vi "Power Output Test Parameters to Stimulus.vi"(10 "PO Test Parameters":T9={"Stimulus"={"Frequency Type"=enum."Band Edges", "Frequency Ranges"=[], "TX 1 Frequency (MHz)"={"Min"=0.0, "Max"=0.0}, "TX 2 Frequency (MHz)"={"Min"=0.0, "Max"=0.0}, "RX Frequency (MHz)"={"Min"=0.0, "Max"=0.0}, "Pad Model Number"="", "Pad Serial Number"="", "Pad Values"=[]}, "Measurement"={"DUT Port"=enum."Port 1", "Direction"=0, "Frequency Step Size"=0}, "Display"={"Frequency"={"Min"=-1.0, "Max"=-1.0}, "Power"={"Min"=-1, "Max"=-1}}, "Limit"={"Min Power (dBm)"=44.0}, "Calibration"={"Calibrated?"=FALSE}} {"Measurement"."Frequency Step Size" items=["0.2", "0.4", "1.0", "2.0", "4.0"]; "Measurement"."Direction" items=["Reverse", "Forward", "Auxiliary"]}) -> (2 "PIM Measurement Stimulus":T1={"Carrier Frequencies"={"C1 Freq, MHz"=0.0, "C2 Freq, MHz"=0.0}, "Carrier Powers"={"C1 Power,dBm"=0.0, "C2 Power, dBm"=0.0}, "Measurement Parameters"={"IM Order"=0, "Averaging"=1, "Direction"=0, "Enable ALC?"=FALSE, "Enable SingleIM?"=FALSE, "Display Units"=enum."dBm", "VA Hold?"=FALSE, "DUT PORT"=enum."Port 1"}, "Measurement Setup"={"Meas Type"=enum."Time", "TXStep"=0}} {"Measurement Setup"."TXStep" items=[".2", ".4", "1.0", "2.0"]; "Measurement Parameters"."Direction" items=["Reverse", "Forward", "Auxiliary"]; "Measurement Parameters"."IM Order" items=["3rd", "5th", "7th", "9th", "11th", "13th", "15th", "17th", "19th", "21st", "23rd", "25th", "27th", "29th", "31st", "33rd"]; "Measurement Parameters"."Averaging" items=["None", "Minimum", "Normal", "High", "Maximum"]})   [LabVIEW 2011]
uses:
  TypeDefs/Power Output Test Parameters.ctl
  TypeDefs/Power Output Stimulus Parameters.ctl
  TypeDefs/Power Output Measurement Parameters.ctl
  BPIMCore EXT/HW IO/DUTport.ctl
  BPIMCore EXT/HW IO/MeasMode.ctl
  BPIMCore EXT/HW IO/PIM Sweep Step Size.ctl
  TypeDefs/Power Output Display Parameters.ctl
  TypeDefs/Power Output Limit Parameters.ctl
  TypeDefs/Power Output Calibration State.ctl
  drivers/PIM/PIM Stimulus.ctl
  drivers/PIM/PIM Cmd Params.ctl
  BPIMCore EXT/HW IO/IMOrder.ctl
  BPIMCore EXT/HW IO/HW Averaging.ctl
  BPIMCore EXT/Display/display_unit_format.ctl
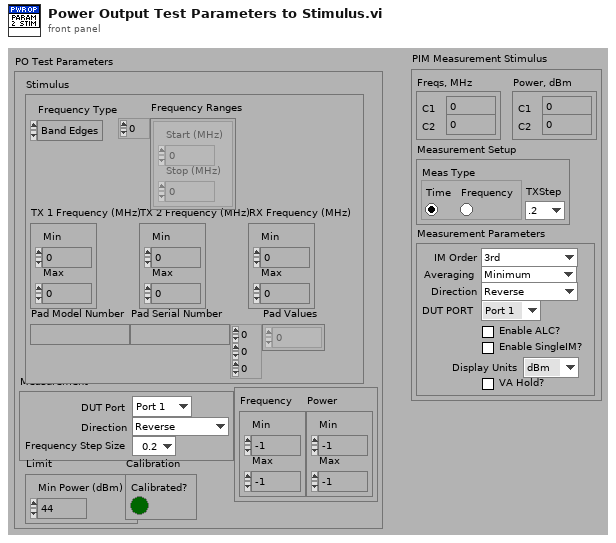
[diagram p1: front panel]
types:
  T1 = typedef "PIM Stimulus.ctl" = cluster{"Carrier Frequencies":cluster{"C1 Freq, MHz":dbl, "C2 Freq, MHz":dbl}, "Carrier Powers":cluster{"C1 Power,dBm":dbl, "C2 Power, dBm":dbl}, "Measurement Parameters":T2, "Measurement Setup":cluster{"Meas Type":enum32{"Time", "Frequency"}, "TXStep":T8}}
  T2 = typedef "PIM Cmd Params.ctl" = cluster{"IM Order":T3, "Averaging":T4, "Direction":T5, "Enable ALC?":bool, "Enable SingleIM?":bool, "Display Units":T6, "VA Hold?":bool, "DUT PORT":T7}
  T3 = typedef "IMOrder.ctl" = u8
  T4 = typedef "HW Averaging.ctl" = u16
  T5 = typedef "MeasMode.ctl" = u16
  T6 = typedef "display_unit_format.ctl" = enum16{"dBm", "dBc"}
  T7 = typedef "DUTport.ctl" = enum16{"Port 1", "Port 2"}
  T8 = typedef "PIM Sweep Step Size.ctl" = u16
  T9 = typedef "Power Output Test Parameters.ctl" = cluster{"Stimulus":T10, "Measurement":T11, "Display":T12, "Limit":T13, "Calibration":T14}
  T10 = typedef "Power Output Stimulus Parameters.ctl" = cluster{"Frequency Type":enum16{"Band Edges", "Custom"}, "Frequency Ranges":cluster{"Start (MHz)":dbl, "Stop (MHz)":dbl}[], "TX 1 Frequency (MHz)":cluster{"Min":dbl, "Max":dbl}, "TX 2 Frequency (MHz)":cluster{"Min":dbl, "Max":dbl}, "RX Frequency (MHz)":cluster{"Min":dbl, "Max":dbl}, "Pad Model Number":string, "Pad Serial Number":string, "Pad Values":dbl[][][]}
  T11 = typedef "Power Output Measurement Parameters.ctl" = cluster{"DUT Port":T7, "Direction":T5, "Frequency Step Size":T8}
  T12 = typedef "Power Output Display Parameters.ctl" = cluster{"Frequency":cluster{"Min":dbl, "Max":dbl}, "Power":cluster{"Min":i32, "Max":i32}}
  T13 = typedef "Power Output Limit Parameters.ctl" = cluster{"Min Power (dBm)":dbl}
  T14 = typedef "Power Output Calibration State.ctl" = cluster{"Calibrated?":bool}
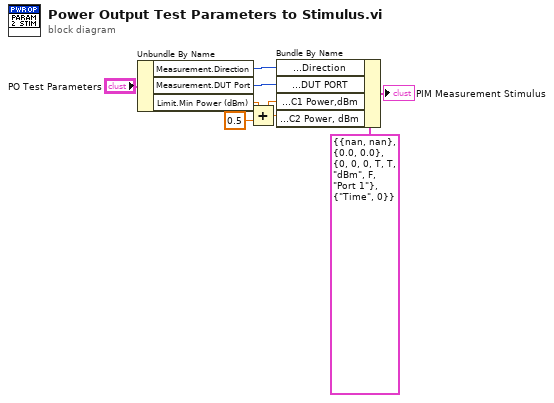
[diagram p0: block diagram]
diagram:
  n1 = Unbundle By Name("PO Test Parameters") -> ("Measurement.Direction"=w6:T5, "Measurement.DUT Port"=w4:T7, "Limit.Min Power (dBm)"=w2:dbl)
  n2 = Add(x=w2, y=0.5) -> (x+y=w1:dbl)
  n3 = Bundle By Name(cluster=T1 {"Carrier Frequencies"={"C1 Freq, MHz"=nan, "C2 Freq, MHz"=nan}, "Carrier Powers"={"C1 Power,dBm"=0.0, "C2 Power, dBm"=0.0}, "Measurement Parameters"={"IM Order"=0, "Averaging"=0, "Direction"=0, "Enable ALC?"=TRUE, "Enable SingleIM?"=TRUE, "Display Units"=enum."dBm", "VA Hold?"=FALSE, "DUT PORT"=enum."Port 1"}, "Measurement Setup"={"Meas Type"=enum."Time", "TXStep"=0}} ("Stimulus"), "Measurement Parameters.Direction"=w6, "Measurement Parameters.DUT PORT"=w4, "Carrier Powers.C1 Power,dBm"=w1, "Carrier Powers.C2 Power, dBm"=w1) -> (→"PIM Measurement Stimulus":T1)
